vi "EXPONENT VALUE (SubVI).vi"(4 "Multiplier":T1) -> (1 "Exponent":dbl)   [LabVIEW 2018]
uses:
  Multiplier.ctl
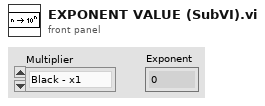
[diagram p1: front panel]
types:
  T1 = typedef "Multiplier.ctl" = enum16{"Black - x1", "Brown - x10", "Red - x100", "Orange - x1.000", "Yellow - x10.000", "Green - x100.000", "Blue - x1.000.000", "Violet -  x 10.000.000", "Grey - x100.000.000", "White - x1.000.000.000", "Silver x - 0,01", "Gold x - 0,1"}
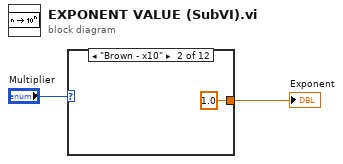
[diagram p0: block diagram]
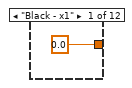
[diagram p2: hidden frame]
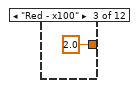
[diagram p3: hidden frame]
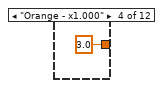
[diagram p4: hidden frame]
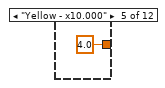
[diagram p5: hidden frame]
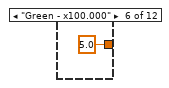
[diagram p6: hidden frame]
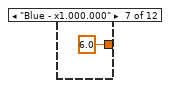
[diagram p7: hidden frame]
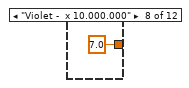
[diagram p8: hidden frame]
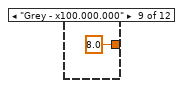
[diagram p9: hidden frame]
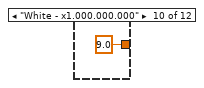
[diagram p10: hidden frame]
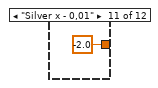
[diagram p11: hidden frame]
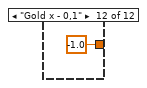
[diagram p12: hidden frame]
diagram:
  n1 = case shown="\"Brown - x10\"" "Multiplier" {
    tunnel: [0.0 1.0 2.0 3.0 4.0 5.0 6.0 7.0 8.0 9.0 -2.0 -1.0] -> w1
    frame "Black - x1" {
    }
    frame "Brown - x10" {
    }
    frame "Red - x100" {
    }
    frame "Orange - x1.000" {
    }
    frame "Yellow - x10.000" {
    }
    frame "Green - x100.000" {
    }
    frame "Blue - x1.000.000" {
    }
    frame "Violet -  x 10.000.000" {
    }
    frame "Grey - x100.000.000" {
    }
    frame "White - x1.000.000.000" {
    }
    frame "Silver x - 0,01" {
    }
    frame "Gold x - 0,1" {
    }
  }
  "Exponent" <- w1
